vi "Replace Item in Tree.vi"(8 "error in":errorcluster, 10 "Active VI Previous State":refnum<class "Standard VI Type.lvclass">, 11 "Module Data":T1) -> (0 "error out":errorcluster, 3 "Module Data":T1)   [LabVIEW 2020, in "Peek Window.lvlib"]
uses:
  Peek Window.lvlib
  MHL Data Cluster.ctl
  VI Types/Standard VI Type/Standard VI Type.lvclass
  VI Types/Standard VI Type/Standard VI Type.lvclass/Standard VI Type.ctl
  VI Types/Standard VI Type/Read Full Qualified Name.vi
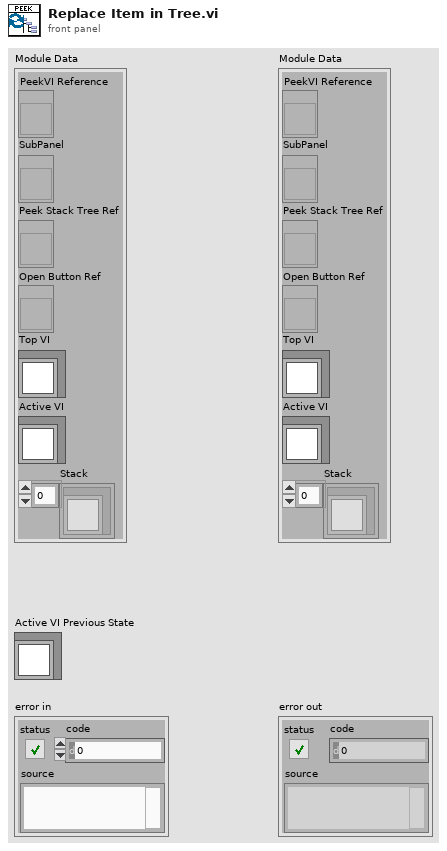
[diagram p1: front panel]
types:
  T1 = typedef "Peek Window.lvlib/MHL Data Cluster.ctl" = cluster{"PeekVI Reference":refnum<vi>, "SubPanel":refnum<vi>, "Peek Stack Tree Ref":refnum<vi>, "Open Button Ref":refnum<vi>, "Top VI":refnum<class "Standard VI Type.lvclass">, "Active VI":refnum<class "Standard VI Type.lvclass">, "Stack":refnum<class "Standard VI Type.lvclass">[]}
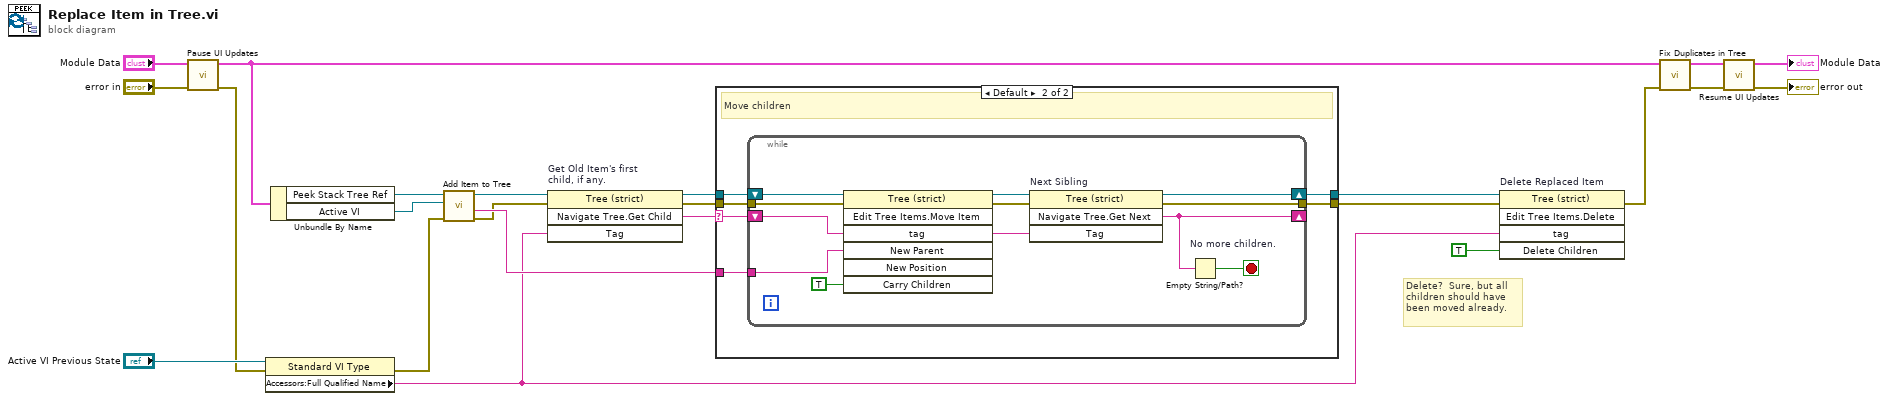
[diagram p0: block diagram]
diagram:
  # "Delete?  Sure, but all children should have been moved already."
  n1 = call "Pause UI Updates.vi"("error in"="error in", "Module Data"="Module Data") -> ("error out"=w5:errorcluster, "Module Data"=w12:T1)  [unwired: 8 in]
  n2 = property class="Standard VI Type"(reference="Active VI Previous State", error in=w5) -> (error out=w4:errorcluster, "Accessors:Full Qualified Name"=w6:string)  [unwired: 1 out]
  n3 = Unbundle By Name(w12) -> ("Peek Stack Tree Ref"=w11:refnum<vi>, "Active VI"=w3:refnum<class "Standard VI Type.lvclass">)
  n4 = call-dynamic "Add Item to Tree.vi"("error in (no error)"=w4, "Standard VI Type in"=w3, "Tree Ref in"=w11) -> ("error out"=w8:errorcluster, "Added Tag"=w9:string, "Tree Ref out"=w10:refnum<vi>)  [unwired: 5 in, 1 out]
  n5 = invoke on="Get Old Item's first\nchild, if any." class="Tree (strict)" method="Navigate Tree.Get Child"(reference=w10, error in=w8, "Tag"=w6) -> (reference out=w22:refnum<vi>, error out=w7:errorcluster, "Navigate Tree:Get Child"=w21:string)  [unwired: 1 in, 1 out]
  n6 = case shown="Default" w21 {
    selector: w21 -> [_ w28]
    tunnel: w7 -> [w24 w31]
    tunnel: w9 -> [_ w30]
    tunnel: w22 -> [w25 w29]
    tunnel: [w24 w27] -> w19
    tunnel: [w25 w26] -> w20
    frame "False" {
      # "No children"
    }
    frame Default {
      # "Move children"
      n7 = while {
        tunnel: w31 -> [w40]
        shift-right: [w33] -> w26
        shift-left: w29 -> [w41]
        tunnel: w30 -> [w42]
        shift-right: [w34] -> _
        shift-left: w28 -> [w36]
        tunnel: [w32] -> w27
        stop <- w35 stop-if-true
        n8 = invoke class="Tree (strict)" method="Edit Tree Items.Move Item"(reference=w41, error in=w40, "tag"=w36, "New Parent"=w42, "Carry Children"=TRUE) -> (reference out=w38:refnum<vi>, error out=w37:errorcluster)  [unwired: 2 in, 5 out]
        n9 = invoke on="Next Sibling" class="Tree (strict)" method="Navigate Tree.Get Next"(reference=w38, error in=w37, "Tag"=w36) -> (reference out=w33:refnum<vi>, error out=w32:errorcluster, "Navigate Tree:Get Next Item"=w34:string)  [unwired: 1 in, 1 out]
        n10 = Empty String/Path? "No more children."(string/path=w34) -> (empty?=w35:bool)
      }
    }
  }
  n11 = invoke on="Delete Replaced Item" class="Tree (strict)" method="Edit Tree Items.Delete"(reference=w20, error in=w19, "tag"=w6, "Delete Children"=TRUE) -> (error out=w2:errorcluster)  [unwired: 1 in, 4 out]
  n12 = call "Fix Duplicates in Tree.vi"("error in (no error)"=w2, "Data in"=w12) -> ("error out"=w1:errorcluster, "Data out"=w15:T1)  [unwired: 8 in]
  n13 = call "Resume UI Updates.vi"("error in"=w1, "Module Data"=w15) -> ("error out"=→"error out":errorcluster, "Module Data"=→"Module Data":T1)  [unwired: 8 in]
